vi "AVL string (SubVI).vi"(2 "error in":errorcluster, 3 "String":string="$$B2359772033694416|AA$GPRMC,155606.000,A,0253.0515,S,07900.7371,W,0.00,,010113,,,A*75|03.8|01.4|03.6|000000000000|20130101155604|14091207|00000000|27F532CB|0000|0.0000|0040|EC53") -> (0 "error out":errorcluster, 1 "Datos":T1)   [LabVIEW 2012]
doc: "VI developed by Juan Andres Valverde\njuandres_valverde@hotmail.com\njuandres.valverde@facebook.com"
panel:
  out "after substring":string
  out "after substring":string
  out "GPRMC":string
  out "Evento":string
  out "before substring":string
  out "Imei":string
  out "CRC(substring)":string
  out "substring CRC":string
  out "size":u32
  out "length":i32
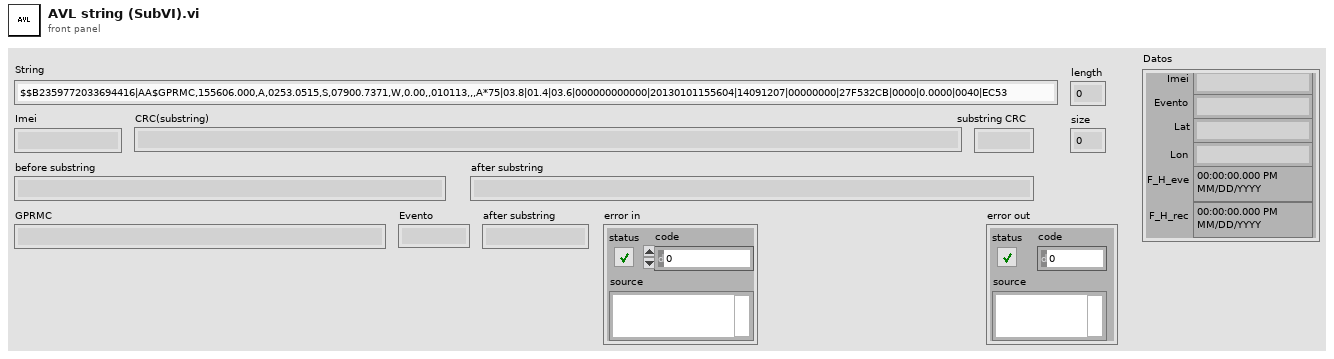
[diagram p1: front panel]
types:
  T1 = cluster{"Imei":string, "Evento":string, "Lat":string, "Lon":string, "F_H_eve":timestamp, "F_H_rec":timestamp}
  T2 = cluster{"Lattitude":string, "Longitude":string, "Speed":dbl, "Track (deg)":dbl}
  T3 = cluster{"before match":string, "before match":string, "Lattitude":string, "Longitude":string, timestamp, "seconds since 1Jan1904":timestamp}
  T4 = typedef "LVDateTimeRec.ctl" = cluster{"fractional second":dbl, "second":i32, "minute":i32, "hour":i32, "day of month":i32, "month":i32, "year":i32, "day of week":i32, "day of year":i32, "DST":i32}
  T5 = cluster{"trimmed string":string, string, "Lattitude":string, "Longitude":string, timestamp, "seconds since 1Jan1904":timestamp}
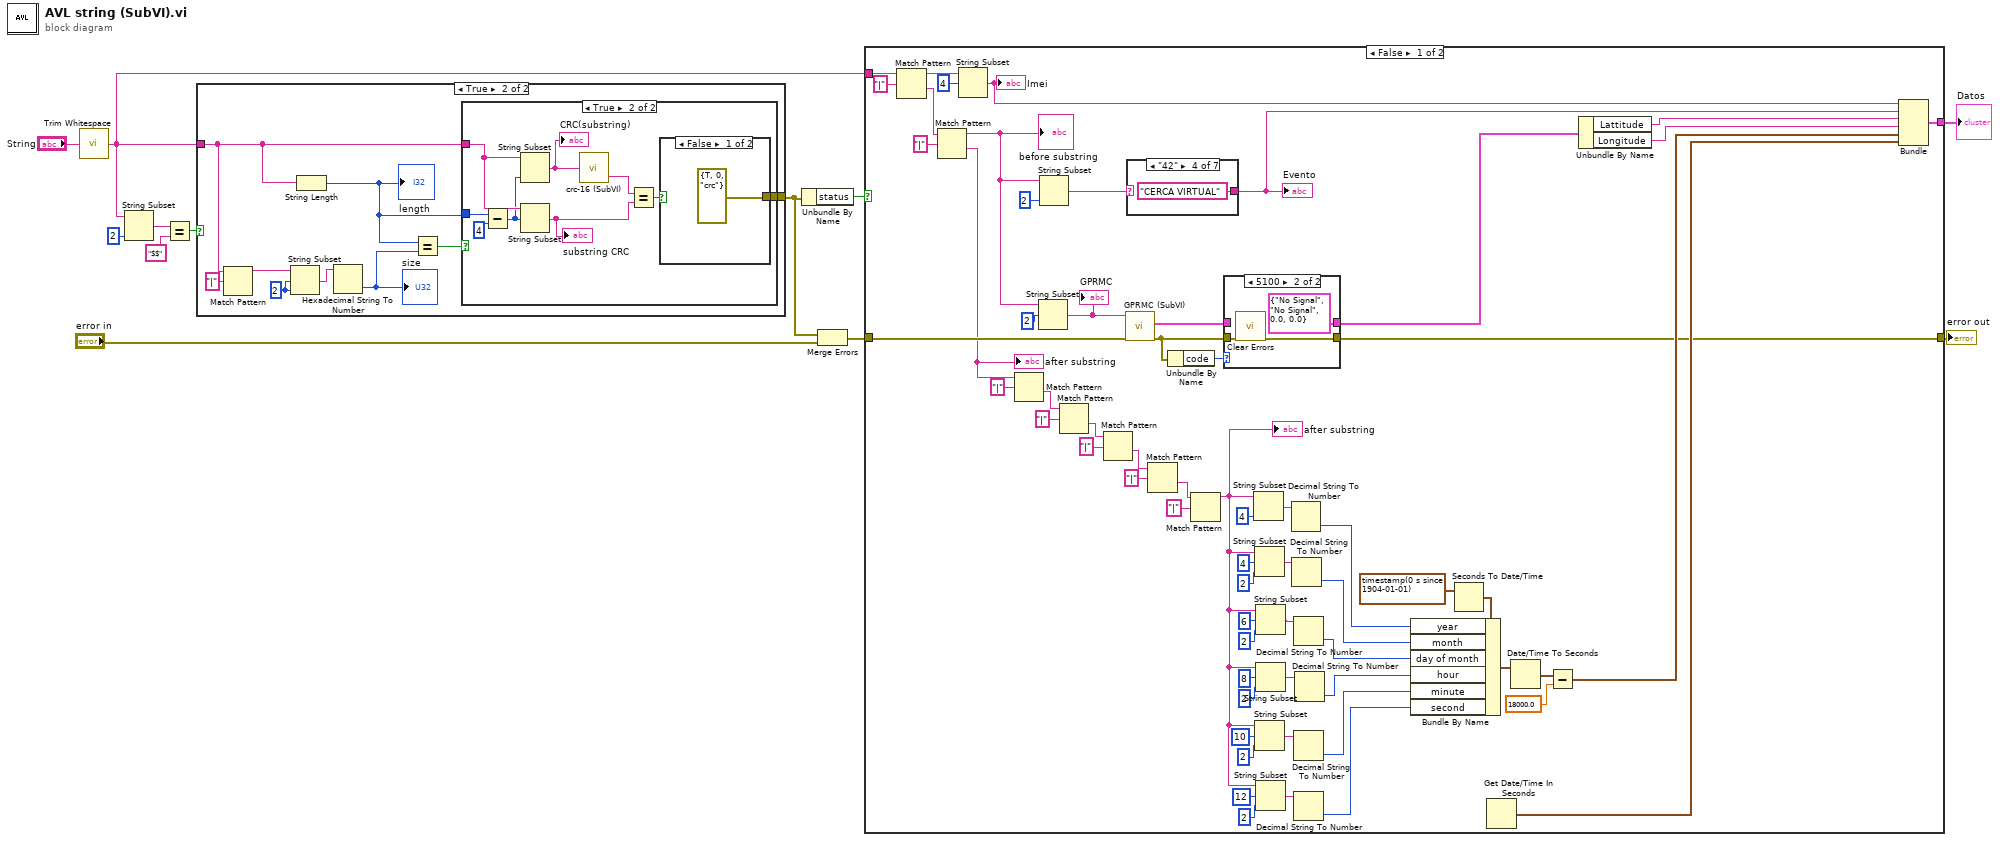
[diagram p0: block diagram]
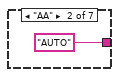
[diagram p3: hidden frame]
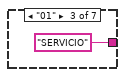
[diagram p4: hidden frame]
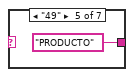
[diagram p5: hidden frame]
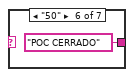
[diagram p6: hidden frame]
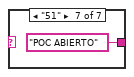
[diagram p7: hidden frame]
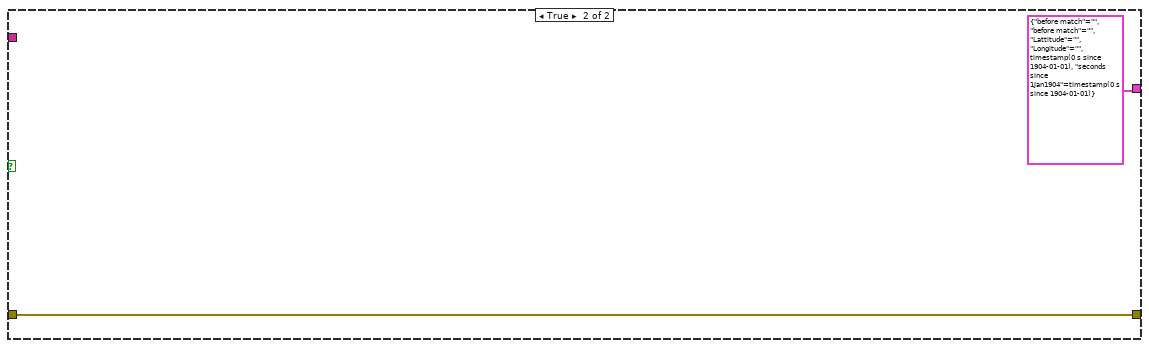
[diagram p9: hidden frame]
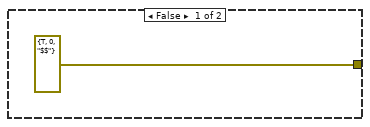
[diagram p10: hidden frame]
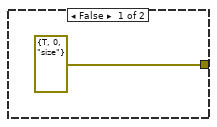
[diagram p11: hidden frame]
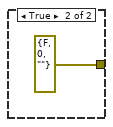
[diagram p12: hidden frame]
diagram:
  n1 = call <vilib>:"Trim Whitespace.vi"("string"="String") -> ("trimmed string"=w2:string)  [unwired: 1 in]
  n2 = String Subset(string=w2, length (rest)=2 ("length (rest)")) -> (substring=w11:string)  [unwired: 1 in]
  n3 = Equal?(x=w11, y="$$") -> (x = y?=w9:bool)
  n4 = case shown="True" w9 {
    tunnel: w2 -> [_ w16]
    tunnel: [errorcluster {"status"=TRUE, "code"=0, "source"="$$"} ("error constant") w14] -> w5
    frame False {
    }
    frame True {
      w21 = 2 ("length (rest)")
      n5 = Match Pattern(string=w16, regular expression="|" ("search string")) -> (before substring=w20:string)  [unwired: 1 in, 3 out]
      n6 = String Subset(string=w20, offset (0)=w21, length (rest)=w21) -> (substring=w19:string)
      n7 = String Length(string=w16) -> (length=w15:i32)
      "length" <- w15
      n8 = Hexadecimal String To Number(string=w19) -> (number=w18:u32)  [unwired: 2 in, 1 out]
      "size" <- w18
      n9 = Equal?(x=w15, y=w18) -> (x = y?=w17:bool)
      n10 = case shown="True" w17 {
        tunnel: w16 -> [_ w30]
        tunnel: w15 -> [_ w31]
        tunnel: [errorcluster {"status"=TRUE, "code"=0, "source"="size"} ("error constant") w24] -> w14
        frame False {
        }
        frame True {
          n11 = Subtract(x=w31, y=u8 4) -> (x-y=w29:i32)
          n12 = String Subset(string=w30, length (rest)=w29) -> (substring=w28:string)  [unwired: 1 in]
          "CRC(substring)" <- w28
          n13 = String Subset(string=w30, offset (0)=w29) -> (substring=w26:string)  [unwired: 1 in]
          "substring CRC" <- w26
          n14 = call "crc-16 (SubVI).vi"("String"=w28) -> ("hex integer string"=w27:string)  [unwired: 1 out]
          n15 = Equal?(x=w27, y=w26) -> (x = y?=w25:bool)
          n16 = case shown="False" w25 {
            tunnel: [errorcluster {"status"=TRUE, "code"=0, "source"="crc"} ("error constant") errorcluster {"status"=FALSE, "code"=0, "source"=""} ("error constant")] -> w24
            frame False {
            }
            frame True {
            }
          }
        }
      }
    }
  }
  n17 = Unbundle By Name(w5) -> ("status"=w8:bool)
  n18 = Merge Errors(w5, "error in") -> (w6:errorcluster)
  n19 = case shown="False" w8 {
    tunnel: w2 -> [w96 _]
    tunnel: w6 -> [w87 w111]
    tunnel: [w38 w111] -> w7
    tunnel: [w44 T3 {"before match"="", "before match"="", "Lattitude"="", "Longitude"="", timestamp(0 s since 1904-01-01), "seconds since 1Jan1904"=timestamp(0 s since 1904-01-01)}] -> w3
    frame False {
      n20 = Match Pattern(string=w96, regular expression="|" ("search string")) -> (before substring=w95:string, after substring=w92:string)  [unwired: 1 in, 2 out]
      n21 = Match Pattern(string=w92, regular expression="|" ("search string")) -> (before substring=w90:string, after substring=w85:string)  [unwired: 1 in, 2 out]
      "before substring" <- w90
      "after substring" <- w85
      n22 = String Subset(string=w95, offset (0)=4) -> (substring=w47:string)  [unwired: 1 in]
      "Imei" <- w47
      n23 = Match Pattern(string=w85, regular expression="|" ("search string")) -> (after substring=w83:string)  [unwired: 1 in, 3 out]
      n24 = String Subset(string=w90, offset (0)=2) -> (substring=w88:string)  [unwired: 1 in]
      "GPRMC" <- w88
      n25 = String Subset(string=w90, length (rest)=2 ("offset (0)")) -> (substring=w36:string)  [unwired: 1 in]
      n26 = Match Pattern(string=w83, regular expression="|" ("search string")) -> (after substring=w79:string)  [unwired: 1 in, 3 out]
      n27 = Match Pattern(string=w79, regular expression="|" ("search string")) -> (after substring=w82:string)  [unwired: 1 in, 3 out]
      n28 = call "GPRMC (SubVI).vi"("error in"=w87, "$GPRMC String In"=w88) -> ("error out"=w39:errorcluster, "LAt Long Spd Tck"=w40:T2)  [unwired: 6 in, 2 out]
      n29 = case shown="\"42\"" w36 {
        selector: w36 -> [w98 _ _ _ _ _ _]
        tunnel: [w98 "AUTO" "SERVICIO" "CERCA VIRTUAL" "PRODUCTO" "POC CERRADO" "POC ABIERTO"] -> w35
        frame "00", Default {
        }
        frame "AA" {
        }
        frame "01" {
        }
        frame "42" {
        }
        frame "49" {
        }
        frame "50" {
        }
        frame "51" {
        }
      }
      "Evento" <- w35
      n30 = Match Pattern(string=w82, regular expression="|" ("search string")) -> (after substring=w77:string)  [unwired: 1 in, 3 out]
      n31 = Unbundle By Name(w39) -> ("code"=w41:i32)
      n32 = Match Pattern(string=w77, regular expression="|" ("search string")) -> (before substring=w48:string)  [unwired: 1 in, 3 out]
      "after substring" <- w48
      n33 = case shown="5100" w41 {
        tunnel: w40 -> [w105 _]
        tunnel: w39 -> [w106 w109]
        tunnel: [w106 w108] -> w38
        tunnel: [w105 T2 {"Lattitude"="No Signal", "Longitude"="No Signal", "Speed"=0.0, "Track (deg)"=0.0} ("LAt Long Spd Tck")] -> w37
        frame 0, Default {
        }
        frame 5100 {
          n34 = call <vilib>:"Clear Errors.vi"("error in (no error)"=w109) -> ("error out"=w108:errorcluster)  [unwired: 6 in]
        }
      }
      n35 = String Subset(string=w48, length (rest)=4 ("length (rest)")) -> (substring=w62:string)  [unwired: 1 in]
      n36 = String Subset(string=w48, offset (0)=4 ("length (rest)"), length (rest)=2 ("length (rest)")) -> (substring=w63:string)
      n37 = String Subset(string=w48, offset (0)=10 ("length (rest)"), length (rest)=2 ("length (rest)")) -> (substring=w66:string)
      n38 = String Subset(string=w48, offset (0)=6 ("length (rest)"), length (rest)=2 ("length (rest)")) -> (substring=w64:string)
      n39 = String Subset(string=w48, offset (0)=8 ("length (rest)"), length (rest)=2 ("length (rest)")) -> (substring=w65:string)
      n40 = String Subset(string=w48, offset (0)=12 ("length (rest)"), length (rest)=2 ("length (rest)")) -> (substring=w67:string)
      n41 = Decimal String To Number(string=w62) -> (number=w69:i32)  [unwired: 2 in, 1 out]
      n42 = Decimal String To Number(string=w63) -> (number=w70:i32)  [unwired: 2 in, 1 out]
      n43 = Decimal String To Number(string=w64) -> (number=w71:i32)  [unwired: 2 in, 1 out]
      n44 = Decimal String To Number(string=w66) -> (number=w73:i32)  [unwired: 2 in, 1 out]
      n45 = Decimal String To Number(string=w67) -> (number=w68:i32)  [unwired: 2 in, 1 out]
      n46 = Decimal String To Number(string=w65) -> (number=w72:i32)  [unwired: 2 in, 1 out]
      n47 = Seconds To Date/Time(time stamp (now)=timestamp(0 s since 1904-01-01) ("time stamp")) -> (date time rec=w61:T4)  [unwired: 1 in]
      n48 = Bundle By Name(cluster=w61, "year"=w69, "month"=w70, "day of month"=w71, "hour"=w72, "minute"=w73, "second"=w68) -> (w75:T4)
      n49 = Get Date/Time In Seconds() -> (seconds since 1Jan1904=w42:timestamp)
      n50 = Date/Time To Seconds(2:w75) -> (0:w76:timestamp)  [unwired: 1 in]
      n51 = Subtract(x=w76, y=18000.0) -> (x-y=w43:timestamp)
      n52 = Unbundle By Name(w37) -> ("Lattitude"=w46:string, "Longitude"=w45:string)
      n53 = Bundle("trimmed string"=w47, w35, "Lattitude"=w46, "Longitude"=w45, w43, "seconds since 1Jan1904"=w42) -> (w44:T5)  [unwired: 1 in]
    }
    frame True {
    }
  }
  "error out" <- w7
  "Datos" <- w3
